vi "Main menu_2_test2.vi"() -> ()   [LabVIEW 2021]
uses:
  <vilib>/event_ctls.llb/lveventtype.ctl
  <vilib>/Utility/file.llb/Write Delimited Spreadsheet (DBL).vi
panel:
  out "Close":bool
  in  "Close app":bool
  out "Waveform Graph 2":waveform(sgl)(graph)
  in  "?":enum32{"Plot", "Control", "Config", "Message"}(tab)
  in  "New plot":bool
  in  "Multicolumn Listbox":i32(listbox)
  in  "Close All plots":bool
  in  "CSV":bool
  in  "Start":bool
  in  "Refresh time (ms)":i32
  in  "Mode":enum32{"Item 0", "Item 1"}(radio)
  in  "Size bytes":i32
  in  "Trace names":string(combo)
  out "IP Free?":bool
  out "Server Ping":string
  out "Saved":bool
  in  "Save conf":bool
  in  "Ping IP":bool
  in  "Port":i32
  in  "hostname":string
  in  "timeout ms":i32
  in  "Send message":bool
  in  "Process 2":i32
  in  "msj":string
  # "hostname: 127.0.0.1\nport: 8085"
  # "hostname\n131.246.75.169"
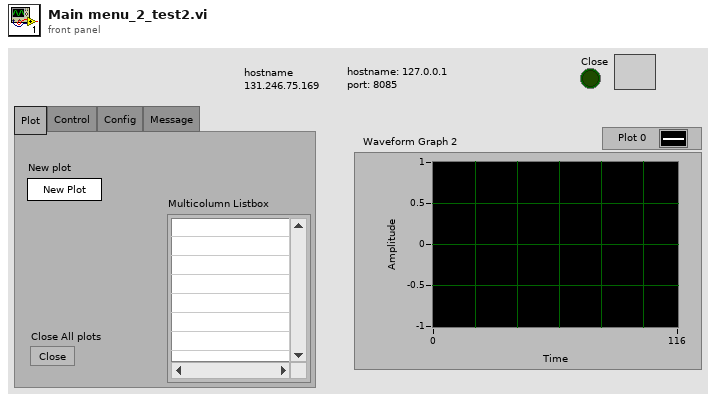
[diagram p1: front panel]
types:
  T1 = cluster{"Port":i32, "hostname":string, "status":bool, "timeout ms":i32, "TRACES_NAMES":string[], "Refresh time ms":i32, "Mode":enum32{"Item 0", "Item 1"}, "Start":bool, "DATA":sgl[][], "SIGNALS_NAMES":string[], "NR_SIGNALS":i32, "NR_TRACES":i32, "ID_TRACE":i32, "Mark":bool, "Counter":i32}
  T2 = enum8{"Enabled", "Disabled", "Disabled and Grayed Out"}
  T3 = typedef "lveventtype.ctl" = enum32{"Null", "Timeout", "Annotation Menu Selection", "Annotation Menu Selection?", "App Instance Close", "App Instance Close?", "Autoscale Range Change", "Bookmark Info Change", "Cell Edit", "Cell Edit?", "Cursor Grab", "Cursor Grab?", "Cursor Menu Selection", "Cursor Menu Selection?", "Cursor Move", "Cursor Release", "Data Change", "Direction Change", "Display State Change", "Drag Ended", "Drag Enter", "Drag Leave", "Drag Over", "Drag Source Update", "Drag Starting", "Drag Starting?", "Drop", "Exec State Change", "Key Down", "Key Down?", "Key Repeat", "Key Repeat?", "Key Up", "Listbox Double Click", "Menu Activation?", "Menu Selection (App)", "Menu Selection? (App)", "Menu Selection (User)", "Mouse Down", "Mouse Down?", "Mouse Enter", "Mouse Leave", "Mouse Move", "Mouse Up", "Mouse Wheel", "NI Security User Change (App)", "Pane Size", "Panel Close", "Panel Close?", "Panel Resize", "Plot Attribute Change", "Scale Range Change", "Shortcut Menu Activation?", "Shortcut Menu Selection (App)", "Shortcut Menu Selection? (App)", "Shortcut Menu Selection (User)", "Tree Double Click", "Tree Drag", "Tree Drag?", "Tree Drop", "Tree Drop?", "Tree Item Close", "Tree Item Close?", "Tree Item Open", "Tree Item Open?", "User Event", "Value Change"}
  T4 = enum16{"open", "replace", "create", "open or create", "replace or create", "replace or create with confirmation"}
  T5 = cluster{"SIZE":i32, "DATA":sgl[], "TRACE_SIZE":i32, "NB_TRACES":i32, "NB_SIGNALS":i32, "string":string[]}
  T6 = enum32{"invalid app kind", "Development System", "Run Time System", "Student Edition", "Embedded LabVIEW", "Evaluation", "Custom"}
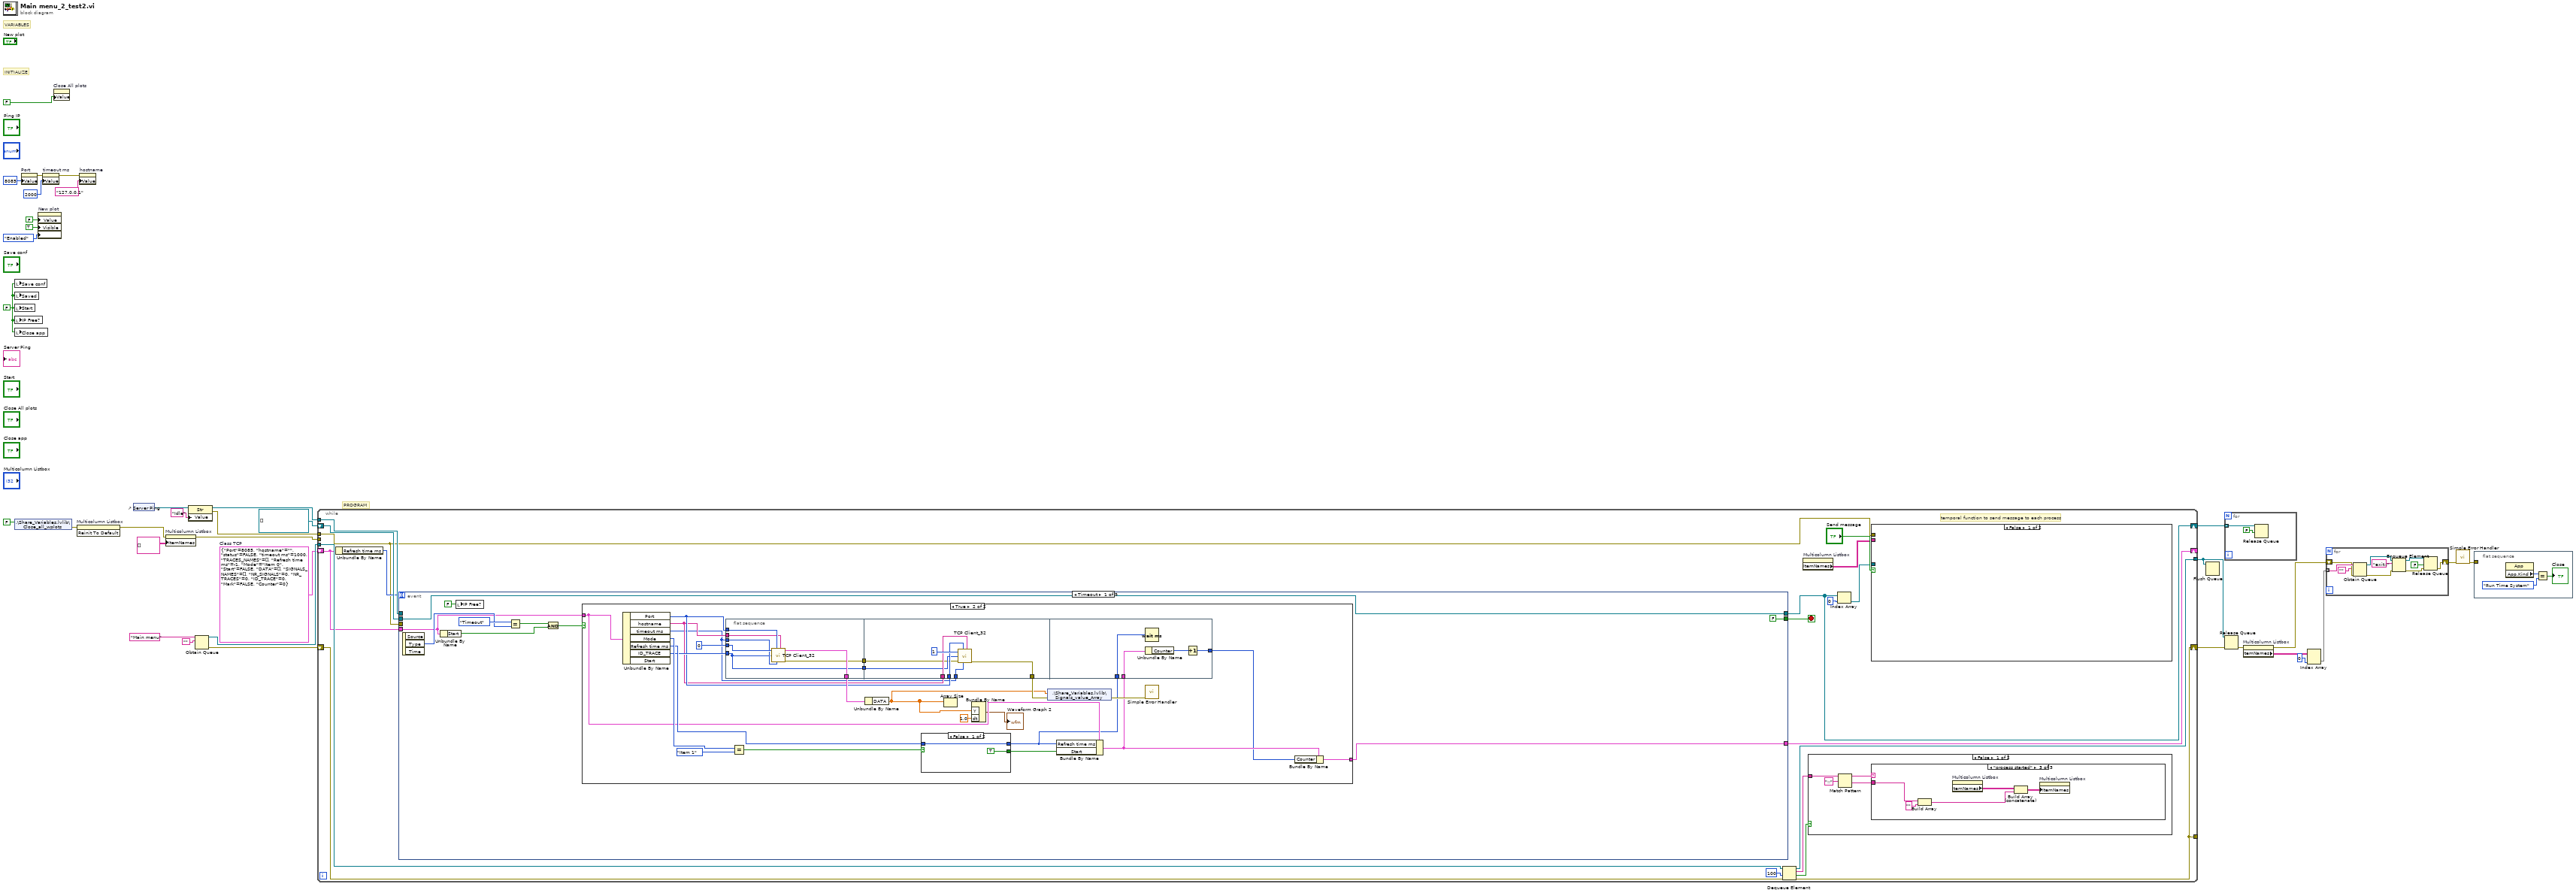
[diagram p0: block diagram]
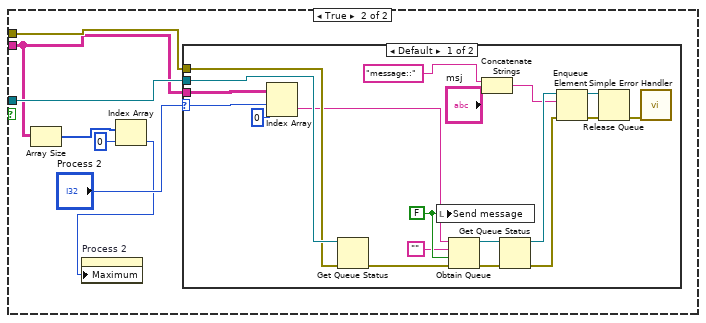
[diagram p2: hidden frame]
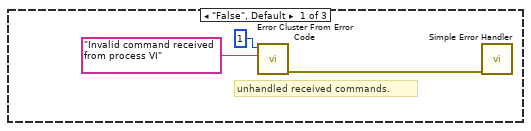
[diagram p4: hidden frame]
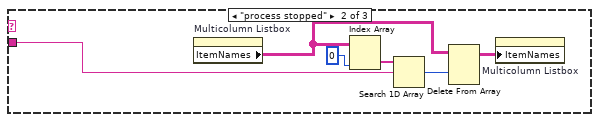
[diagram p5: hidden frame]
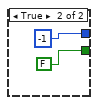
[diagram p8: hidden frame]
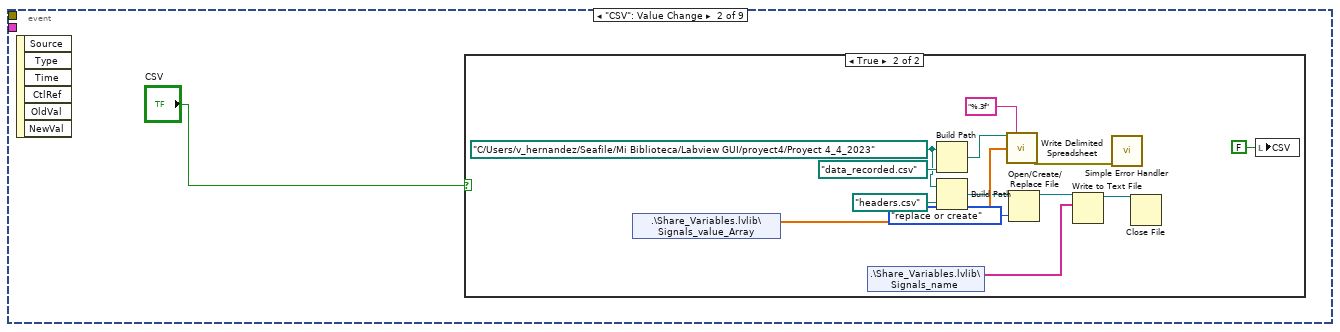
[diagram p9: hidden frame]
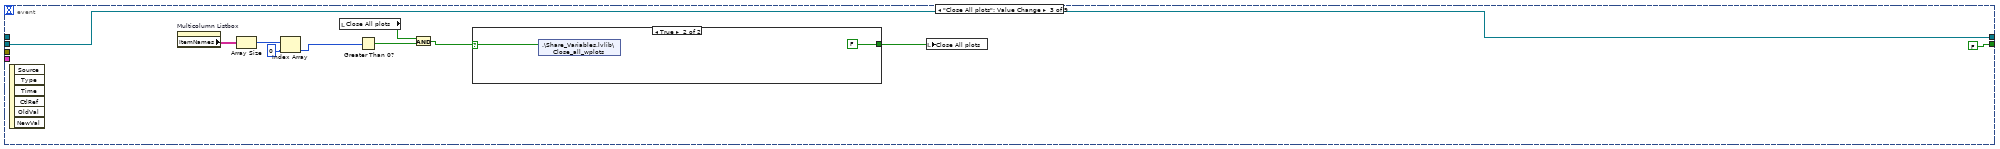
[diagram p11: hidden frame]
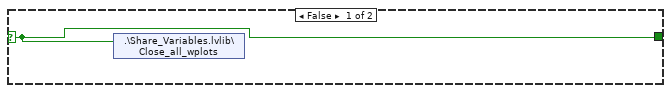
[diagram p12: hidden frame]
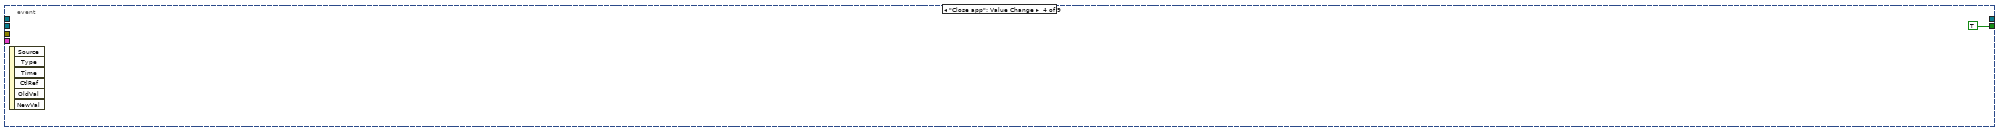
[diagram p13: hidden frame]
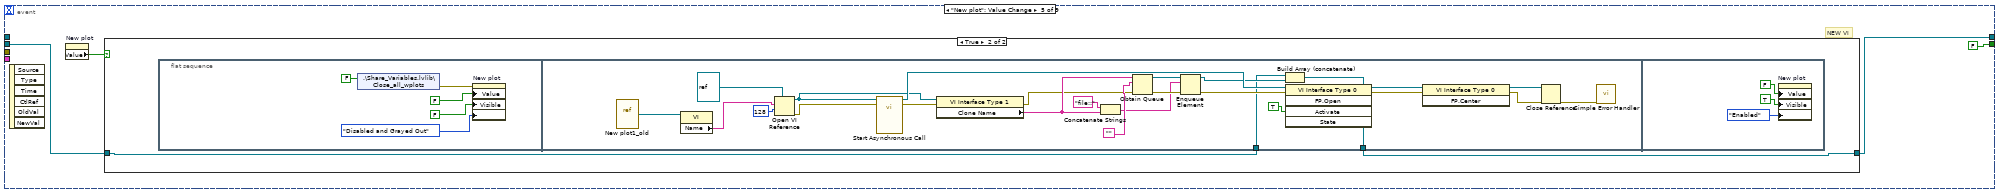
[diagram p14: hidden frame]
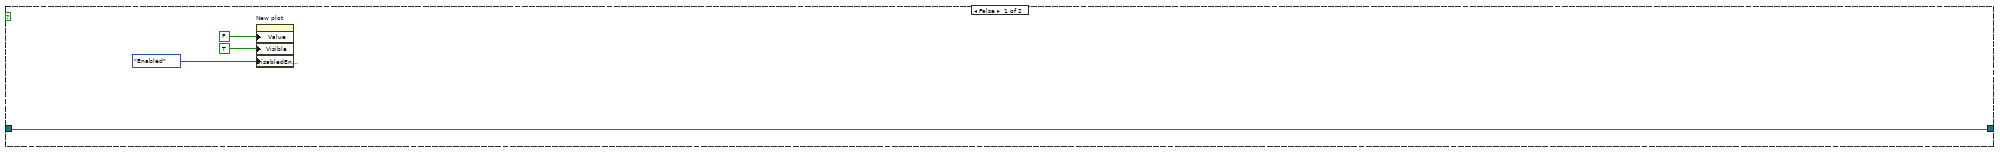
[diagram p15: hidden frame]
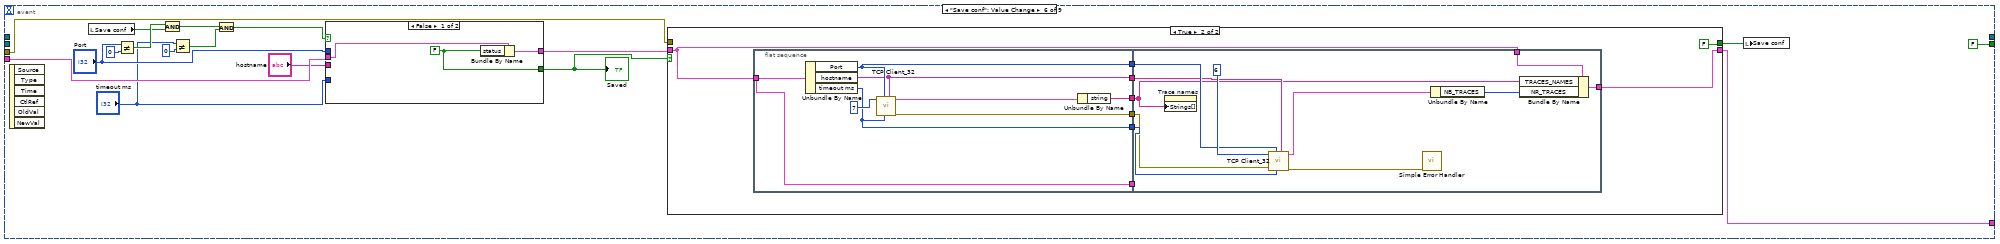
[diagram p16: hidden frame]
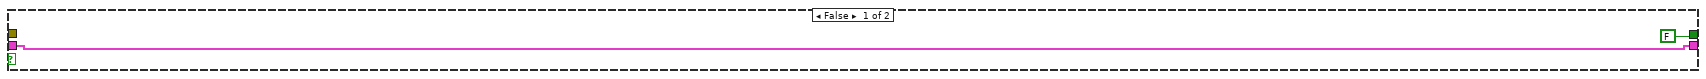
[diagram p17: hidden frame]
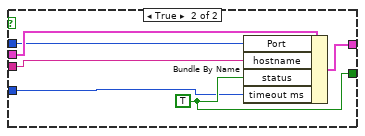
[diagram p18: hidden frame]
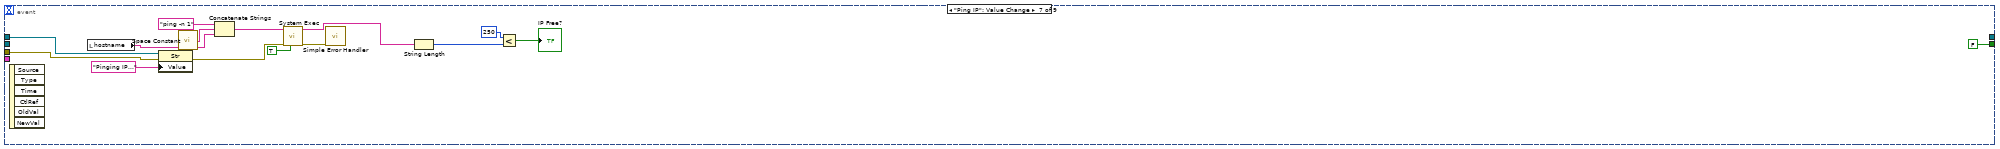
[diagram p19: hidden frame]
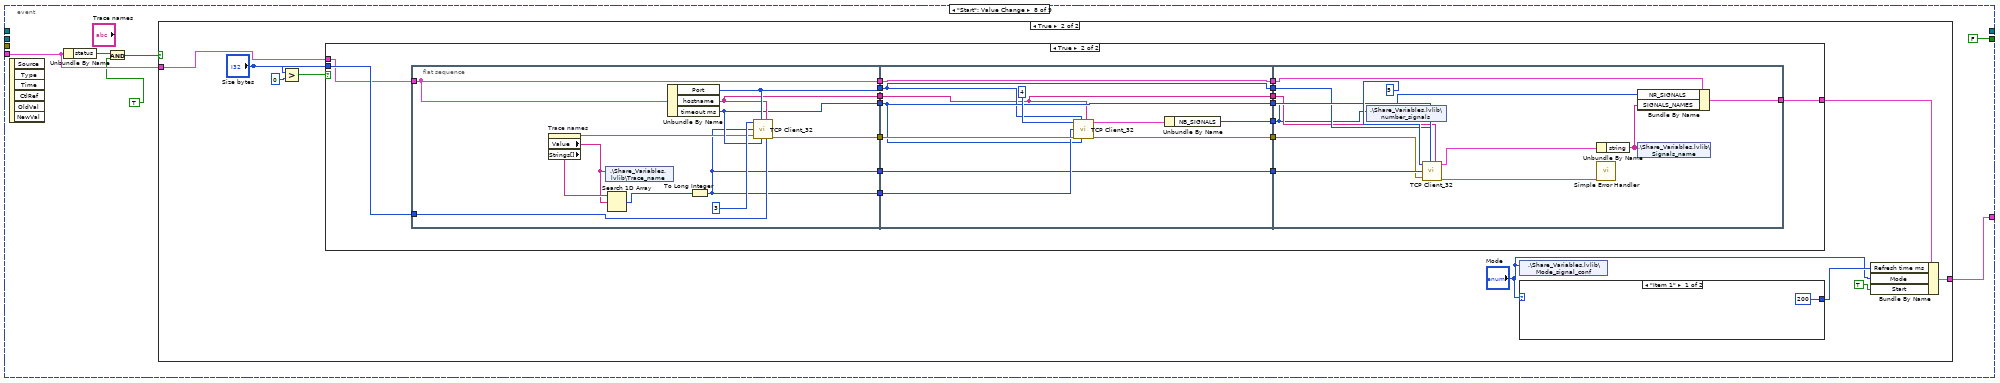
[diagram p20: hidden frame]
diagram:
  w12 = T1 {"Port"=8085, "hostname"="", "status"=FALSE, "timeout ms"=1000, "TRACES_NAMES"=[], "Refresh time ms"=-1, "Mode"=enum."Item 0", "Start"=FALSE, "DATA"=[], "SIGNALS_NAMES"=[], "NR_SIGNALS"=0, "NR_TRACES"=0, "ID_TRACE"=0, "Mark"=FALSE, "Counter"=0}  # Class TCP
  w3 = FALSE ("Save conf")
  # "PROGRAM"
  # "INITIALIZE"
  # "VARIABLES"
  n1 = local write "Save conf"(w3) -> ()
  n2 = local write "Saved"(w3) -> ()
  n3 = local write "Start"(w3) -> ()
  n4 = local write "IP Free?"(w3) -> ()
  n5 = local write "Close app"(w3) -> ()
  n6 = shared-variable ".\\Share_Variables.lvlib\\Close_all_wplots"(FALSE ("Close_all_wplots")) -> (error out=w6:errorcluster)  [unwired: 1 in]
  n7 = property on="Port" class="DigNum (strict)"("Value"=8085) -> (error out=w7:errorcluster)  [unwired: 2 in, 1 out]
  n8 = property on="New plot" class="Bool (strict)"("Value"=FALSE ("New plot"), "Visible"=TRUE, "DisabledEnum"=T2."Enabled" ("Disabled")) -> ()  [unwired: 2 in, 2 out]
  n9 = property on="timeout ms" class="DigNum (strict)"(error in=w7, "Value"=2000 ("timeout ms")) -> (error out=w2:errorcluster)  [unwired: 1 in, 1 out]
  n10 = property on="Close All plots" class="Bool (strict)"("Value"=FALSE ("Cancel Button")) -> ()  [unwired: 2 in, 2 out]
  n11 = invoke on="Multicolumn Listbox" class="MCListbox (strict)" method="Reinit To Default"(error in=w6) -> (error out=w15:errorcluster)  [unwired: 2 in, 2 out]
  n12 = property on="hostname" class="Str"(error in=w2, "Value"="127.0.0.1" ("hostname")) -> ()  [unwired: 1 in, 2 out]
  n13 = control-ref of="Server Ping"() -> (w9:refnum<vi>)
  n14 = property on="Multicolumn Listbox" class="MCListbox (strict)"(error in=w15, "ItemNames"=string[][] [] ("Item Names")) -> (error out=w16:errorcluster)  [unwired: 1 in, 1 out]
  n15 = property class="Str"(reference=w9, "Value"="Idle" ("Ping status")) -> (reference out=w11:refnum<vi>, error out=w10:errorcluster)  [unwired: 1 in]
  n16 = Obtain Queue(name (unnamed)="Main menu", element data type="") -> (queue out=w28:refnum<queue>, error out=w26:errorcluster)  [unwired: 3 in, 1 out]
  n17 = while {
    shift-right: [w37] -> w32
    shift-left: refnum<queue>[] [] -> [w53]
    tunnel: w28 -> [w52]
    tunnel: [w49] -> w18
    shift-right: [w42] -> w27
    shift-left: w26 -> [w48]
    tunnel: w16 -> [_]
    shift-right: [w46] -> _
    shift-left: w12 -> [w44]
    tunnel: w11 -> [w45]
    tunnel: w10 -> [w39]
    tunnel: [w42] -> _
    stop <- w54 stop-if-true
    # "temporal function to send message to each process"
    n18 = Unbundle By Name(w44) -> ("Refresh time ms"=w43:i32)
    n19 = event shown="[0] Timeout" {
      selector: _ -> [_ _ _ _ _ _ _ _ _]
      dyn-events: _ -> [_ _ _ _ _ _ _ _ _]
      timeout: w43 -> [_ _ _ _ _ _ _ _ _]
      tunnel: [FALSE ("f") _ FALSE ("f") TRUE ("f") FALSE ("f") FALSE ("f") FALSE ("f") FALSE ("f") FALSE ("f")] -> w54
      tunnel: [w108 _ w178 _ w185 _ _ _ _] -> w37
      tunnel: w53 -> [w108 _ w178 _ w184 _ _ _ _]
      tunnel: [w100 _ _ _ _ w232 _ w299 _] -> w46
      tunnel: w44 -> [w101 _ _ _ _ w240 _ w300 w382]
      tunnel: w45 -> [_ _ _ _ _ _ w296 _ _]
      tunnel: w39 -> [_ _ _ _ _ w235 w283 _ _]
      event Timeout {
        n20 = event-data() -> ("Type"=w105:T3)  [unwired: 1 in, 2 out]
        n21 = Unbundle By Name(w101) -> ("Start"=w103:bool)
        n22 = local write "IP Free?"(FALSE ("IP Free?")) -> ()
        n23 = Equal?(x=lveventtype."Timeout" ("Type"), y=w105) -> (x = y?=w104:bool)
        n24 = And(x=w104, y=w103) -> (x .and. y?=w102:bool)
        n25 = case shown="True" w102 {
          tunnel: w101 -> [w109 w127]
          tunnel: [w109 w115] -> w100
          frame False {
          }
          frame True {
            n26 = Unbundle By Name(w127) -> ("Port"=w122:i32, "hostname"=w121:string, "timeout ms"=w119:i32, "Mode"=w132:enum32{"Item 0", "Item 1"}, "Refresh time ms"=w129:i32, "ID_TRACE"=w124:i32)  [unwired: 1 out]
            n27 = flat-sequence {
              tunnel: 0 ("CMD") -> [w139]
              tunnel: w122 -> [w138]
              tunnel: w124 -> [w134]
              tunnel: w119 -> [w137]
              tunnel: w121 -> [w136]
              tunnel: [w135] -> w123
              tunnel: [w134] -> w120
              tunnel: [w133] -> w118
              tunnel: w122 -> [w145]
              tunnel: w121 -> [w144]
              tunnel: w120 -> [w143]
              tunnel: w119 -> [w142]
              tunnel: w118 -> [w141]
              tunnel: [w140] -> w117
              tunnel: w116 -> [w150]
              tunnel: [w148] -> w114
              tunnel: w112 -> [w147]
              frame #0 {
                n28 = call "TCP Client_32.vi"("CMD"=w139, "remote port \nor service name"=w138, "ID_Trace"=w134, "timeout ms"=w137, "Address"=w136) -> ("Output cluster"=w135:T5, "error out"=w133:errorcluster)  [unwired: 3 in, 1 out]
              }
              frame #1 {
                n29 = call "TCP Client_32.vi"("CMD"=1, "remote port \nor service name"=w145, "ID_Trace"=w143, "error in (no error)"=w141, "timeout ms"=w142, "Address"=w144) -> ("error out"=w140:errorcluster)  [unwired: 2 in, 2 out]
              }
              frame #2 {
                n30 = Wait (ms)(milliseconds to wait=w147) -> ()  [unwired: 1 out]
                n31 = Unbundle By Name(w150) -> ("Counter"=w149:i32)
                n32 = Increment(x=w149) -> (x+1=w148:i32)
              }
            }
            n33 = Equal?(x=w132, y=enum32{"Item 0", "Item 1"}."Item 1" ("Mode")) -> (x = y?=w130:bool)
            n34 = Unbundle By Name(w123) -> ("DATA"=w110:sgl[])
            n35 = case shown="False" w130 {
              tunnel: [TRUE FALSE] -> w128
              tunnel: [w151 i8 -1 ("t")] -> w112
              tunnel: w129 -> [w151 _]
              frame False {
              }
              frame True {
              }
            }
            n36 = Array Size(array=w110) -> ()  [unwired: 1 out]
            n37 = Bundle By Name("Y"=w110, "dt"=1.0) -> (→"Waveform Graph 2":waveform(sgl))  [unwired: 1 in]
            n38 = shared-variable ".\\Share_Variables.lvlib\\Signals_value_Array"(w110, error in=w117) -> (error out=w126:errorcluster)
            n39 = Bundle By Name(cluster=w127, "Refresh time ms"=w112, "Start"=w128) -> (w116:T1)
            n40 = call <vilib>:"Simple Error Handler.vi"("error in (no error)"=w126) -> ()  [unwired: 4 in, 5 out]
            n41 = Bundle By Name(cluster=w116, "Counter"=w114) -> (w115:T1)
          }
        }
      }
      event "CSV": Value Change {
        n42 = event-data() -> ()  [unwired: 1 in, 6 out]
        n43 = case shown="True" "CSV" {
          frame False {
          }
          frame True {
            w163 = path "C:/Users/v_hernandez/Seafile/Mi Biblioteca/Labview GUI/proyect4/Proyect 4_4_2023" ("base path")
            n44 = shared-variable ".\\Share_Variables.lvlib\\Signals_value_Array"() -> (w165:dbl[])  [unwired: 1 in, 1 out]
            n45 = shared-variable ".\\Share_Variables.lvlib\\Signals_name"() -> (w158:string[])  [unwired: 1 in, 1 out]
            n46 = Build Path(base path=w163, name or relative path=path "data_recorded.csv") -> (appended path=w164:path)
            n47 = Build Path(base path=w163, name or relative path=path "headers.csv") -> (appended path=w161:path)
            n48 = call-poly <vilib>:"Write Delimited Spreadsheet.vi"("file path (dialog if empty)"=w164, "format (%.3f)"="%.3f", "1D data"=w165) -> ("error out"=w166:errorcluster)  [unwired: 11 in, 1 out]
            n49 = Open/Create/Replace File(file path (use dialog)=w161, operation (0:open)=T4."replace or create") -> (refnum out=w159:refnum<file>)  [unwired: 4 in, 2 out]
            n50 = Write to Text File(file (use dialog)=w159, text=w158) -> (refnum out=w157:refnum<file>)  [unwired: 2 in, 2 out]
            n51 = call <vilib>:"Simple Error Handler.vi"("error in (no error)"=w166) -> ()  [unwired: 4 in, 5 out]
            n52 = Close File(refnum=w157) -> ()  [unwired: 1 in, 2 out]
            n53 = local write "CSV"(FALSE ("CSV")) -> ()
          }
        }
      }
      event "Close All plots": Value Change {
        n54 = event-data() -> ()  [unwired: 1 in, 6 out]
        n55 = property on="Multicolumn Listbox" class="MCListbox (strict)"() -> ("ItemNames"=w172:string[][])  [unwired: 2 in, 2 out]
        n56 = Array Size(array=w172) -> (size(s)=w176:i32[])
        n57 = Index Array(array=w176, index=0) -> (element=w174:i32)
        n58 = local read "Close All plots"() -> (w171:bool)
        n59 = Greater Than 0?(x=w174) -> (x > 0?=w169:bool)
        n60 = And(x=w171, y=w169) -> (x .and. y?=w170:bool)
        n61 = case shown="True" w170 {
          selector: w170 -> [w179 w180]
          tunnel: [w179 FALSE] -> w173
          frame False {
            n62 = shared-variable ".\\Share_Variables.lvlib\\Close_all_wplots"(w179) -> ()  [unwired: 1 in, 1 out]
          }
          frame True {
            n63 = shared-variable ".\\Share_Variables.lvlib\\Close_all_wplots"(w180) -> ()  [unwired: 1 in, 1 out]
          }
        }
        n64 = local write "Close All plots"(w173) -> ()
      }
      event "Close app": Value Change {
        n65 = event-data() -> ()  [unwired: 1 in, 6 out]
      }
      event "New plot": Value Change {
        # "NEW VI"
        n66 = event-data() -> ()  [unwired: 1 in, 6 out]
        n67 = property on="New plot" class="Bool (strict)"() -> ("Value"=w186:bool)  [unwired: 2 in, 2 out]
        n68 = case shown="True" w186 {
          tunnel: [w187 w192] -> w185
          tunnel: w184 -> [w187 w191]
          frame False {
            n69 = property on="New plot" class="Bool (strict)"("Value"=FALSE ("New plot"), "Visible"=TRUE, "DisabledEnum"=T2."Enabled" ("Disabled")) -> ()  [unwired: 2 in, 2 out]
          }
          frame True {
            n70 = flat-sequence {
              tunnel: [w203] -> w192
              tunnel: w191 -> [w202]
              frame #0 {
                n71 = shared-variable ".\\Share_Variables.lvlib\\Close_all_wplots"(FALSE ("Close_all_wplots")) -> (error out=w193:errorcluster)  [unwired: 1 in]
                n72 = property on="New plot" class="Bool (strict)"(error in=w193, "Value"=FALSE ("New plot"), "Visible"=FALSE, "DisabledEnum"=T2."Disabled and Grayed Out" ("Disabled")) -> ()  [unwired: 1 in, 2 out]
              }
              frame #1 {
                n73 = vi-ref "New plot1_old.vi"() -> (w216:refnum<vi>)
                n74 = property class="VI"(reference=w216) -> ("Name"=w222:string)  [unwired: 1 in, 2 out]
                n75 = Open VI Reference(type specifier VI Refnum (for type only)=refnum<vi> refnum, vi path=w222, options=128) -> (vi reference=w213:refnum<vi>, error out=w218:errorcluster)  [unwired: 3 in]
                n76 = call-by-ref "Start Asynchronous Call"(reference=w213, error in=w218) -> (reference out=w217:refnum<vi>, error out=w207:errorcluster)  [unwired: 1 in, 1 out]
                n77 = property class="VI Interface Type 1"(reference=w213, error in=w207) -> (error out=w208:errorcluster, "Clone Name"=w210:string)  [unwired: 1 out]
                n78 = Concatenate Strings("file::" ("string"), w210) -> (w201:string)
                n79 = Obtain Queue(name (unnamed)=w210, element data type="", error in (no error)=w208) -> (queue out=w209:refnum<queue>, error out=w206:errorcluster)  [unwired: 2 in, 1 out]
                n80 = Enqueue Element(queue=w209, element=w201, error in (no error)=w206) -> (queue out=w204:refnum<queue>, error out=w205:errorcluster)  [unwired: 1 in, 1 out]
                n81 = Build Array (concatenate)(w202, w204) -> (w203:refnum<queue>[])
                n82 = invoke class="VI Interface Type 0" method="FP.Open"(reference=w217, error in=w205, "Activate"=TRUE ("Activate?")) -> (reference out=w215:refnum<vi>, error out=w200:errorcluster)  [unwired: 2 in, 3 out]
                n83 = invoke class="VI Interface Type 0" method="FP.Center"(reference=w215, error in=w200) -> (reference out=w214:refnum<vi>, error out=w199:errorcluster)  [unwired: 1 in, 1 out]
                n84 = Close Reference(reference=w214, error in (no error)=w199) -> (error out=w198:errorcluster)
                n85 = call <vilib>:"Simple Error Handler.vi"("error in (no error)"=w198) -> ()  [unwired: 4 in, 5 out]
              }
              frame #2 {
                n86 = property on="New plot" class="Bool (strict)"("Value"=FALSE ("Value (Signaling)"), "Visible"=TRUE, "DisabledEnum"=T2."Enabled" ("Disabled")) -> ()  [unwired: 2 in, 2 out]
              }
            }
          }
        }
      }
      event "Save conf": Value Change {
        n87 = event-data() -> ()  [unwired: 1 in, 6 out]
        n88 = local read "Save conf"() -> (w237:bool)
        n89 = Not Equal?(x="Port", y=0) -> (x != y?=w241:bool)
        n90 = And(x=w241, y=w237) -> (x .and. y?=w227:bool)
        n91 = Not Equal?(x="timeout ms", y=0) -> (x != y?=w229:bool)
        n92 = And(x=w227, y=w229) -> (x .and. y?=w228:bool)
        n93 = case shown="False" w228 {
          tunnel: [w273 w278] -> w236
          tunnel: "Port" -> [_ w280]
          tunnel: "hostname" -> [_ w279]
          tunnel: [w275 w276] -> w233
          tunnel: w240 -> [w274 w281]
          tunnel: "timeout ms" -> [_ w277]
          frame False {
            w273 = FALSE
            n94 = Bundle By Name(cluster=w274, "status"=w273) -> (w275:T1)
          }
          frame True {
            w278 = TRUE
            n95 = Bundle By Name(cluster=w281, "Port"=w280, "hostname"=w279, "status"=w278, "timeout ms"=w277) -> (w276:T1)
          }
        }
        "Saved" <- w236
        n96 = case shown="True" w236 {
          tunnel: w235 -> [_ _]
          tunnel: [FALSE FALSE] -> w234
          tunnel: w233 -> [w243 w248]
          tunnel: [w243 w247] -> w232
          frame False {
          }
          frame True {
            n97 = flat-sequence {
              tunnel: [w259] -> w252
              tunnel: w248 -> [w256]
              tunnel: [w258] -> w251
              tunnel: [w257] -> w250
              tunnel: [w256] -> w249
              tunnel: [w255] -> w246
              tunnel: [w254] -> w245
              tunnel: w252 -> [w271]
              tunnel: w251 -> [w270]
              tunnel: w250 -> [w269]
              tunnel: w249 -> [_]
              tunnel: w248 -> [w268]
              tunnel: [w267] -> w247
              tunnel: w246 -> [w263]
              tunnel: w245 -> [w264]
              frame #0 {
                n98 = Unbundle By Name(w256) -> ("Port"=w259:i32, "hostname"=w258:string, "timeout ms"=w257:i32)
                n99 = call "TCP Client_32.vi"("CMD"=7, "remote port \nor service name"=w259, "timeout ms"=w257, "Address"=w258) -> ("Output cluster"=w260:T5, "error out"=w254:errorcluster)  [unwired: 4 in, 1 out]
                n100 = Unbundle By Name(w260) -> ("string"=w255:string[])
              }
              frame #1 {
                n101 = property on="Trace names" class="CmbBox"("Strings[]"=w263) -> ()  [unwired: 2 in, 2 out]
                n102 = call "TCP Client_32.vi"("CMD"=6, "remote port \nor service name"=w271, "error in (no error)"=w264, "timeout ms"=w269, "Address"=w270) -> ("Output cluster"=w266:T5, "error out"=w262:errorcluster)  [unwired: 3 in, 1 out]
                n103 = call <vilib>:"Simple Error Handler.vi"("error in (no error)"=w262) -> ()  [unwired: 4 in, 5 out]
                n104 = Unbundle By Name(w266) -> ("NB_TRACES"=w265:i32)
                n105 = Bundle By Name(cluster=w268, "TRACES_NAMES"=w263, "NR_TRACES"=w265) -> (w267:T1)
              }
            }
          }
        }
        n106 = local write "Save conf"(w234) -> ()
      }
      event "Ping IP": Value Change {
        n107 = event-data() -> ()  [unwired: 1 in, 6 out]
        n108 = local read "hostname"() -> (w291:string)
        n109 = property class="Str"(reference=w296, error in=w283, "Value"="Pinging IP...") -> (error out=w294:errorcluster)  [unwired: 1 out]
        n110 = call <vilib>:"Space Constant.vi"() -> ("String"=w292:string)
        n111 = Concatenate Strings("ping -n 1" ("Value"), w292, w291) -> (w290:string)
        n112 = call <vilib>:"System Exec.vi"("run minimized? (F)"=TRUE, "error in (no error)"=w294, "command line"=w290) -> ("error out"=w284:errorcluster, "standard output"=w288:string)  [unwired: 5 in, 2 out]
        n113 = call <vilib>:"Simple Error Handler.vi"("error in (no error)"=w284) -> ()  [unwired: 4 in, 5 out]
        n114 = String Length(string=w288) -> (length=w289:i32)
        n115 = Less?(x=250, y=w289) -> (x < y?=→"IP Free?":bool)
      }
      event "Start": Value Change {
        n116 = event-data() -> ()  [unwired: 1 in, 6 out]
        n117 = Unbundle By Name(w300) -> ("status"=w302:bool)
        n118 = And(x=w302, y=TRUE) -> (x .and. y?=w301:bool)
        n119 = case shown="True" w301 {
          tunnel: w300 -> [w303 w306]
          tunnel: [w303 w312] -> w299
          frame False {
          }
          frame True {
            n120 = Greater?(x="Size bytes", y=0) -> (0:w308:bool)
            n121 = case shown="True" w308 {
              tunnel: "Size bytes" -> [_ w330]
              tunnel: w306 -> [w313 w329]
              tunnel: [w313 w314] -> w305
              frame False {
              }
              frame True {
                n122 = flat-sequence {
                  tunnel: w330 -> [w342]
                  tunnel: w329 -> [w335]
                  tunnel: [w340] -> w328
                  tunnel: [w339] -> w327
                  tunnel: [w338] -> w326
                  tunnel: [w337] -> w325
                  tunnel: [w334] -> w324
                  tunnel: [w335] -> w323
                  tunnel: [w334] -> w321
                  tunnel: w328 -> [w345]
                  tunnel: w327 -> [w344]
                  tunnel: w326 -> [w346]
                  tunnel: w325 -> [w353]
                  tunnel: w324 -> [w351]
                  tunnel: w323 -> [w349]
                  tunnel: [w349] -> w322
                  tunnel: w321 -> [w348]
                  tunnel: [w348] -> w320
                  tunnel: [w347] -> w319
                  tunnel: [w346] -> w318
                  tunnel: [w345] -> w317
                  tunnel: [w344] -> w316
                  tunnel: [w343] -> w315
                  tunnel: w322 -> [w365]
                  tunnel: w320 -> [w363]
                  tunnel: w319 -> [w362]
                  tunnel: w318 -> [w361]
                  tunnel: w317 -> [w360]
                  tunnel: w316 -> [w359]
                  tunnel: w315 -> [w354]
                  tunnel: [w356] -> w314
                  frame #0 {
                    n123 = property on="Trace names" class="CmbBox"() -> (error out=w336:errorcluster, "Value"=w331:string, "Strings[]"=w333:string[])  [unwired: 2 in, 1 out]
                    n124 = shared-variable ".\\Share_Variables.lvlib\\Trace_name"(w331) -> ()  [unwired: 1 in, 1 out]
                    n125 = Search 1D Array(1D array=w333, element=w331) -> (index of element=w332:i32)  [unwired: 1 in]
                    n126 = Unbundle By Name(w335) -> ("Port"=w340:i32, "hostname"=w339:string, "timeout ms"=w338:i32)
                    n127 = To Long Integer(number=w332) -> (32bit integer=w334:i32)
                    n128 = call "TCP Client_32.vi"("CMD"=3, "remote port \nor service name"=w340, "ID_Trace"=w334, "error in (no error)"=w336, "timeout ms"=w338, "Address"=w339, "TRACE_SIZE"=w342) -> ("error out"=w337:errorcluster)  [unwired: 1 in, 2 out]
                  }
                  frame #1 {
                    n129 = call "TCP Client_32.vi"("CMD"=4, "remote port \nor service name"=w345, "ID_Trace"=w351, "error in (no error)"=w353, "timeout ms"=w346, "Address"=w344) -> ("Output cluster"=w350:T5, "error out"=w347:errorcluster)  [unwired: 2 in, 1 out]
                    n130 = Unbundle By Name(w350) -> ("NB_SIGNALS"=w343:i32)
                  }
                  frame #2 {
                    n131 = shared-variable ".\\Share_Variables.lvlib\\number_signals"(w354) -> ()  [unwired: 1 in, 1 out]
                    n132 = call "TCP Client_32.vi"("CMD"=5, "remote port \nor service name"=w360, "ID_Trace"=w363, "error in (no error)"=w362, "timeout ms"=w361, "Address"=w359) -> ("Output cluster"=w357:T5, "error out"=w358:errorcluster)  [unwired: 2 in, 1 out]
                    n133 = Unbundle By Name(w357) -> ("string"=w355:string[])
                    n134 = call <vilib>:"Simple Error Handler.vi"("error in (no error)"=w358) -> ()  [unwired: 4 in, 5 out]
                    n135 = Bundle By Name(cluster=w365, "NR_SIGNALS"=w354, "SIGNALS_NAMES"=w355) -> (w356:T1)
                    n136 = shared-variable ".\\Share_Variables.lvlib\\Signals_name"(w355) -> ()  [unwired: 1 in, 1 out]
                  }
                }
              }
            }
            n137 = shared-variable ".\\Share_Variables.lvlib\\Mode_signal_conf"("Mode") -> ()  [unwired: 1 in, 1 out]
            n138 = case shown="\"Item 1\"" "Mode" {
              tunnel: [200 ("Refresh time (sec)") w367] -> w310
              frame "Item 1" {
              }
              frame "Item 0", Default {
                n139 = Multiply(x=1, y="Refresh time (ms)") -> (x*y=w367:i32)
              }
            }
            n140 = Bundle By Name(cluster=w305, "Refresh time ms"=w310, "Mode"="Mode", "Start"=TRUE) -> (w312:T1)
          }
        }
      }
      event "Trace names": Value Change {
        n141 = event-data() -> ()  [unwired: 1 in, 6 out]
        n142 = property on="Trace names" class="CmbBox"() -> ("Value"=w374:string, "Strings[]"=w373:string[])  [unwired: 2 in, 2 out]
        n143 = Search 1D Array(1D array=w373, element=w374) -> (index of element=w372:i32)  [unwired: 1 in]
        n144 = Unbundle By Name(w382) -> ("Port"=w380:i32, "hostname"=w379:string, "timeout ms"=w378:i32)
        n145 = To Long Integer(number=w372) -> (32bit integer=w371:i32)
        n146 = call "TCP Client_32.vi"("CMD"=2, "remote port \nor service name"=w380, "ID_Trace"=w371, "timeout ms"=w378, "Address"=w379) -> ("Output cluster"=w377:T5, "error out"=w375:errorcluster)  [unwired: 3 in, 1 out]
        n147 = call <vilib>:"Simple Error Handler.vi"("error in (no error)"=w375) -> ()  [unwired: 4 in, 5 out]
        n148 = Unbundle By Name(w377) -> ("TRACE_SIZE"=w376:i32)
        n149 = property on="Size bytes" class="DigNum (strict)"("Value"=w376) -> ()  [unwired: 2 in, 2 out]
      }
    }
    n150 = Dequeue Element(queue=w52, timeout in ms (-1)=100, error in (no error)=w48) -> (queue out=w49:refnum<queue>, element=w51:string, timed out?=w50:bool, error out=w42:errorcluster)
    n151 = property on="Multicolumn Listbox" class="MCListbox (strict)"() -> ("ItemNames"=w40:string[][])  [unwired: 2 in, 2 out]
    n152 = case shown="False" w50 {
      tunnel: w51 -> [w83 _]
      frame False {
        n153 = Match Pattern(string=w83, regular expression="::") -> (before substring=w82:string, after substring=w81:string)  [unwired: 1 in, 2 out]
        n154 = case shown="\"process started\"" w82 {
          tunnel: w81 -> [_ w93 w98]
          frame "False", Default {
            # "unhandled received commands."
            n155 = call <vilib>:"Error Cluster From Error Code.vi"("error message (\"\")"="Invalid command received from process VI" ("error message (\"\")"), "error code (0)"=1) -> ("error out"=w85:errorcluster)  [unwired: 7 in]
            n156 = call <vilib>:"Simple Error Handler.vi"("error in (no error)"=w85) -> ()  [unwired: 4 in, 5 out]
          }
          frame "process stopped" {
            n157 = property on="Multicolumn Listbox" class="MCListbox (strict)"() -> ("ItemNames"=w89:string[][])  [unwired: 2 in, 2 out]
            n158 = Index Array(array=w89, index (col)=0 ("disabled index (col)")) -> (element=w90:string[])  [unwired: 1 in]
            n159 = Search 1D Array(1D array=w90, element=w93) -> (index of element=w91:i32)  [unwired: 1 in]
            n160 = Delete From Array(array=w89, index (row)=w91) -> (array with subset deleted=w88:string[][])  [unwired: 2 in, 1 out]
            n161 = property on="Multicolumn Listbox" class="MCListbox (strict)"("ItemNames"=w88) -> ()  [unwired: 2 in, 2 out]
          }
          frame "process started" {
            n162 = Build Array(w98, "" ("element")) -> (w96:string[])
            n163 = property on="Multicolumn Listbox" class="MCListbox (strict)"() -> ("ItemNames"=w95:string[][])  [unwired: 2 in, 2 out]
            n164 = Build Array (concatenate)(w95, w96) -> (w94:string[][])
            n165 = property on="Multicolumn Listbox" class="MCListbox (strict)"("ItemNames"=w94) -> ()  [unwired: 2 in, 2 out]
          }
        }
      }
      frame True {
      }
    }
    n166 = Index Array(array=w37, index=0) -> (element=w36:refnum<queue>)
    n167 = case shown="False" "Send message" {
      tunnel: w40 -> [_ w58]
      tunnel: w39 -> [_ w60]
      tunnel: w36 -> [_ w59]
      frame False {
      }
      frame True {
        n168 = Array Size(array=w58) -> (size(s)=w56:i32[])
        n169 = Index Array(array=w56, index=0) -> (element=w55:i32)
        n170 = property on="Process 2" class="DigNum (strict)"("Maximum"=w55) -> ()  [unwired: 2 in, 2 out]
        n171 = case shown="Default" "Process 2" {
          selector: "Process 2" -> [w78 _]
          tunnel: w58 -> [w80 _]
          tunnel: w60 -> [w68 _]
          tunnel: w59 -> [w69 _]
          frame Default {
            w64 = FALSE ("create if not found? (T)")
            n172 = Index Array(array=w80, index (row)=w78, index (col)=0 ("disabled index (col)")) -> (element=w62:string)
            n173 = Get Queue Status(queue=w69, error in (no error)=w68) -> (error out=w66:errorcluster)  [unwired: 1 in, 7 out]
            n174 = local write "Send message"(w64) -> ()
            n175 = Obtain Queue(name (unnamed)=w62, element data type="", create if not found? (T)=w64, error in (no error)=w66) -> (queue out=w67:refnum<queue>, error out=w65:errorcluster)  [unwired: 1 in, 1 out]
            n176 = Concatenate Strings("message::", "msj") -> (w73:string)
            n177 = Get Queue Status(queue=w67, error in (no error)=w65) -> (queue out=w77:refnum<queue>, error out=w76:errorcluster)  [unwired: 1 in, 6 out]
            n178 = Enqueue Element(queue=w77, element=w73, error in (no error)=w76) -> (queue out=w72:refnum<queue>, error out=w71:errorcluster)  [unwired: 1 in, 1 out]
            n179 = Release Queue(queue=w72, error in (no error)=w71) -> (error out=w70:errorcluster)  [unwired: 1 in, 2 out]
            n180 = call <vilib>:"Simple Error Handler.vi"("error in (no error)"=w70) -> ()  [unwired: 4 in, 5 out]
          }
          frame ..-1 {
          }
        }
      }
    }
  }
  n181 = Flush Queue(queue=w18) -> ()  [unwired: 1 in, 3 out]
  n182 = for {
    tunnel: w32 -> [w384] mode=indexing
    n183 = Release Queue(queue=w384, force destroy? (F)=FALSE) -> ()  [unwired: 1 in, 3 out]
  }
  n184 = Release Queue(queue=w18, error in (no error)=w27) -> (error out=w25:errorcluster)  [unwired: 1 in, 2 out]
  n185 = property on="Multicolumn Listbox" class="MCListbox (strict)"(error in=w25) -> (error out=w21:errorcluster, "ItemNames"=w24:string[][])  [unwired: 1 in, 1 out]
  n186 = Index Array(array=w24, index (col)=0 ("disabled index (col)")) -> (element=w22:string[])  [unwired: 1 in]
  n187 = for {
    tunnel: w22 -> [w394] mode=indexing
    shift-right: [w391] -> w20
    shift-left: w21 -> [w393]
    n188 = Obtain Queue(name (unnamed)=w394, element data type="", error in (no error)=w393) -> (queue out=w386:refnum<queue>, error out=w388:errorcluster)  [unwired: 2 in, 1 out]
    n189 = Enqueue Element(queue=w386, element="exit::", error in (no error)=w388) -> (queue out=w385:refnum<queue>, error out=w387:errorcluster)  [unwired: 1 in, 1 out]
    n190 = Release Queue(queue=w385, force destroy? (F)=FALSE, error in (no error)=w387) -> (error out=w391:errorcluster)  [unwired: 2 out]
  }
  n191 = call <vilib>:"Simple Error Handler.vi"("error in (no error)"=w20) -> ("error out"=w19:errorcluster)  [unwired: 4 in, 4 out]
  n192 = flat-sequence {
    tunnel: w19 -> [_]
    frame #0 {
      n193 = property class="App"() -> ("App.Kind"=w397:T6)  [unwired: 2 in, 2 out]
      n194 = Equal?(x=w397, y=T6."Run Time System" ("Application:Kind")) -> (x = y?=→"Close":bool)
    }
  }
